vi "System@ParameterRead__Parameter.vi"(1 "ParamterIn":string) -> (0 "ParamterOut":string)   [LabVIEW 2019]
uses:
  MainFrame/Global.vi
panel:
  in  "FileName":string(combo)
  in  "Confirm":bool
  # "System@ParameterRead $ParameterFile"
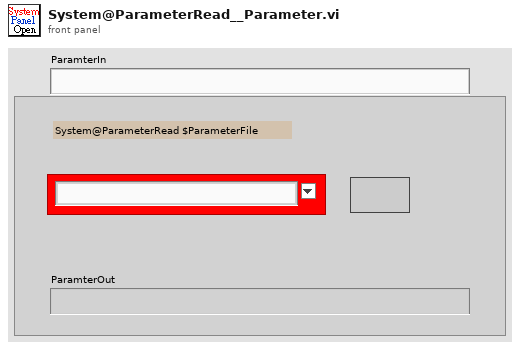
[diagram p1: front panel]
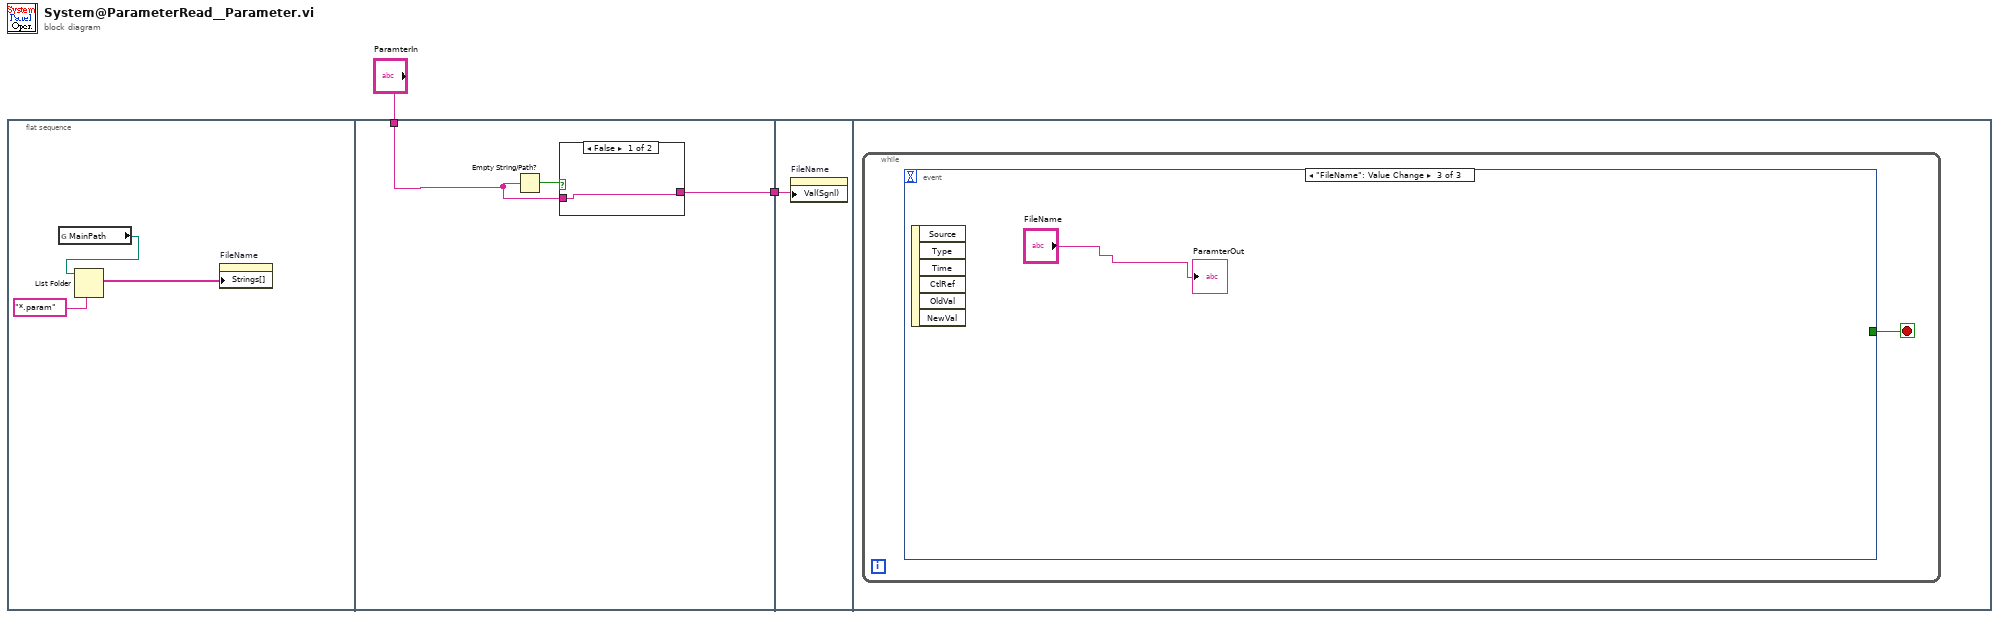
[diagram p0: block diagram]
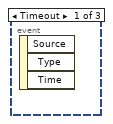
[diagram p3: hidden frame]
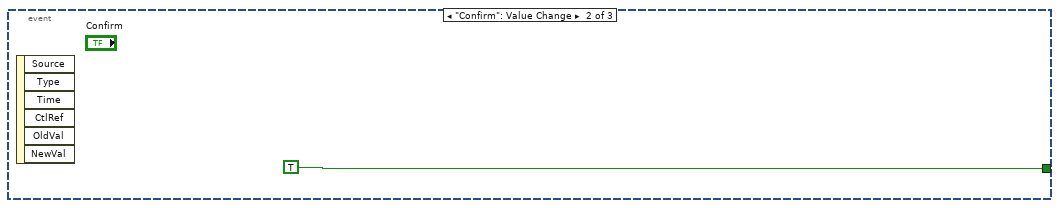
[diagram p4: hidden frame]
diagram:
  n1 = flat-sequence {
    tunnel: "ParamterIn" -> [w6]
    tunnel: [w7] -> w1
    tunnel: w1 -> [w11]
    frame #0 {
      n2 = global read "Global.vi" "MainPath"() -> (w5:path)
      n3 = List Folder(path=w5, pattern="*.param") -> (filenames=w3:string[])  [unwired: 2 in, 3 out]
      n4 = property on="FileName" class="CmbBox"("Strings[]"=w3) -> ()  [unwired: 2 in, 2 out]
    }
    frame #1 {
      n5 = Empty String/Path?(string/path=w6) -> (empty?=w8:bool)
      n6 = case shown="False" w8 {
        tunnel: w6 -> [w9 w10]
        tunnel: [w9 w10] -> w7
        frame False {
        }
        frame True {
        }
      }
    }
    frame #2 {
      n7 = property on="FileName" class="CmbBox"("Val(Sgnl)"=w11) -> ()  [unwired: 2 in, 2 out]
    }
    frame #3 {
      n8 = while {
        stop <- w12 stop-if-true
        n9 = event shown="[2] \"FileName\": Value Change" {
          selector: _ -> [_ _ _]
          dyn-events: _ -> [_ _ _]
          timeout: _ -> [_ _ _]
          tunnel: [_ TRUE _] -> w12
          event Timeout {
            n10 = event-data() -> ()  [unwired: 1 in, 3 out]
          }
          event "Confirm": Value Change {
            n11 = event-data() -> ()  [unwired: 1 in, 6 out]
          }
          event "FileName": Value Change {
            n12 = event-data() -> ()  [unwired: 1 in, 6 out]
            "ParamterOut" <- "FileName"
          }
        }
      }
    }
  }
